vi "Generator.vi"() -> (2 "Y":dbl[](array[numeric]))   [LabVIEW 2025]
uses:
  <vilib>/measure/NI_MABase.lvlib
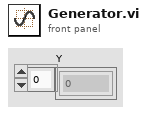
[diagram p1: front panel]
types:
  T1 = enum16{"Sine Wave", "Triangle Wave", "Square Wave", "Sawtooth Wave"}
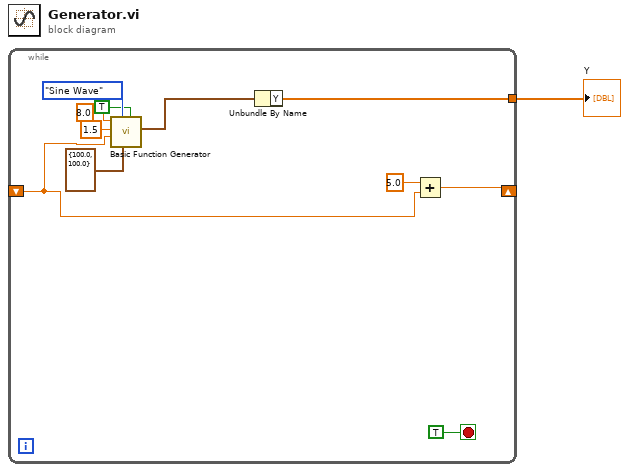
[diagram p0: block diagram]
diagram:
  n1 = while {
    shift-right: [w8] -> _
    shift-left: _ -> [w6]
    tunnel: [w2] -> w1
    stop <- TRUE stop-if-true
    # "UDP Multicast Sender Loop"
    n2 = call <vilib>:"Basic Function Generator.vi"("reset signal"=TRUE, "sampling info"=cluster{"Fs":dbl, "#s":dbl} {"Fs"=100.0, "#s"=100.0}, "signal type"=T1."Sine Wave", "phase"=w6, "amplitude"=1.5, "frequency"=8.0) -> ("signal out"=w3:waveform(dbl))  [unwired: 3 in, 2 out]
    n3 = Unbundle By Name(w3) -> ("Y"=w2:dbl[])
    n4 = Add(x=5.0, y=w6) -> (x+y=w8:dbl)
  }
  "Y" <- w1
